vi "find_stage_goal_pose.vi"(6 "Pivot point (mm)":dbl[](array[numeric]), 7 "G^A: Goal (ASAP)":T1, 9 "L^A: Light pose (ASAP)":T1, 10 "E^B: current stage pose (base)":T1, 11 "O^A: base Orientation (ASAP)":T1) -> (1 "E'^B: goal pose (Base)":T1, 2 "t^O: translation ASAP -> base":T1, 3 "L^P: rotation of lights (Pivot)":T1)   [LabVIEW 2013]
uses:
  <vilib>/Analysis/Matrix/Datatypes/RealMatrix.ctl
  <vilib>/Analysis/baseanly.llb/Real A x B.vi
  <vilib>/Analysis/Matrix/Numeric/Conversions/Array To Matrix - RA.vi
  <vilib>/Analysis/NI_AALBase.lvlib
  <vilib>/Analysis/Matrix/NI_Matrix.lvlib
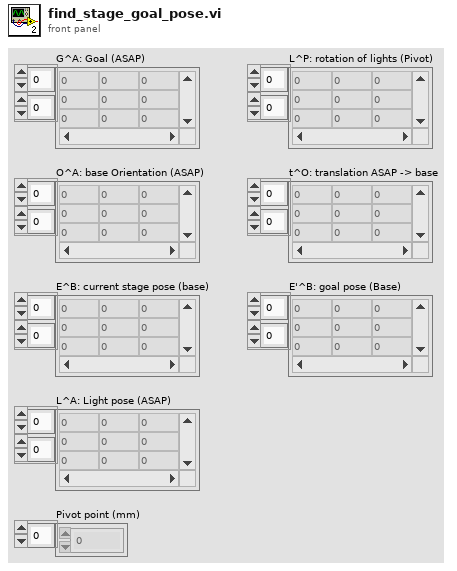
[diagram p1: front panel]
types:
  T1 = typedef "NI_Matrix.lvlib/RealMatrix.ctl" = dbl[][]
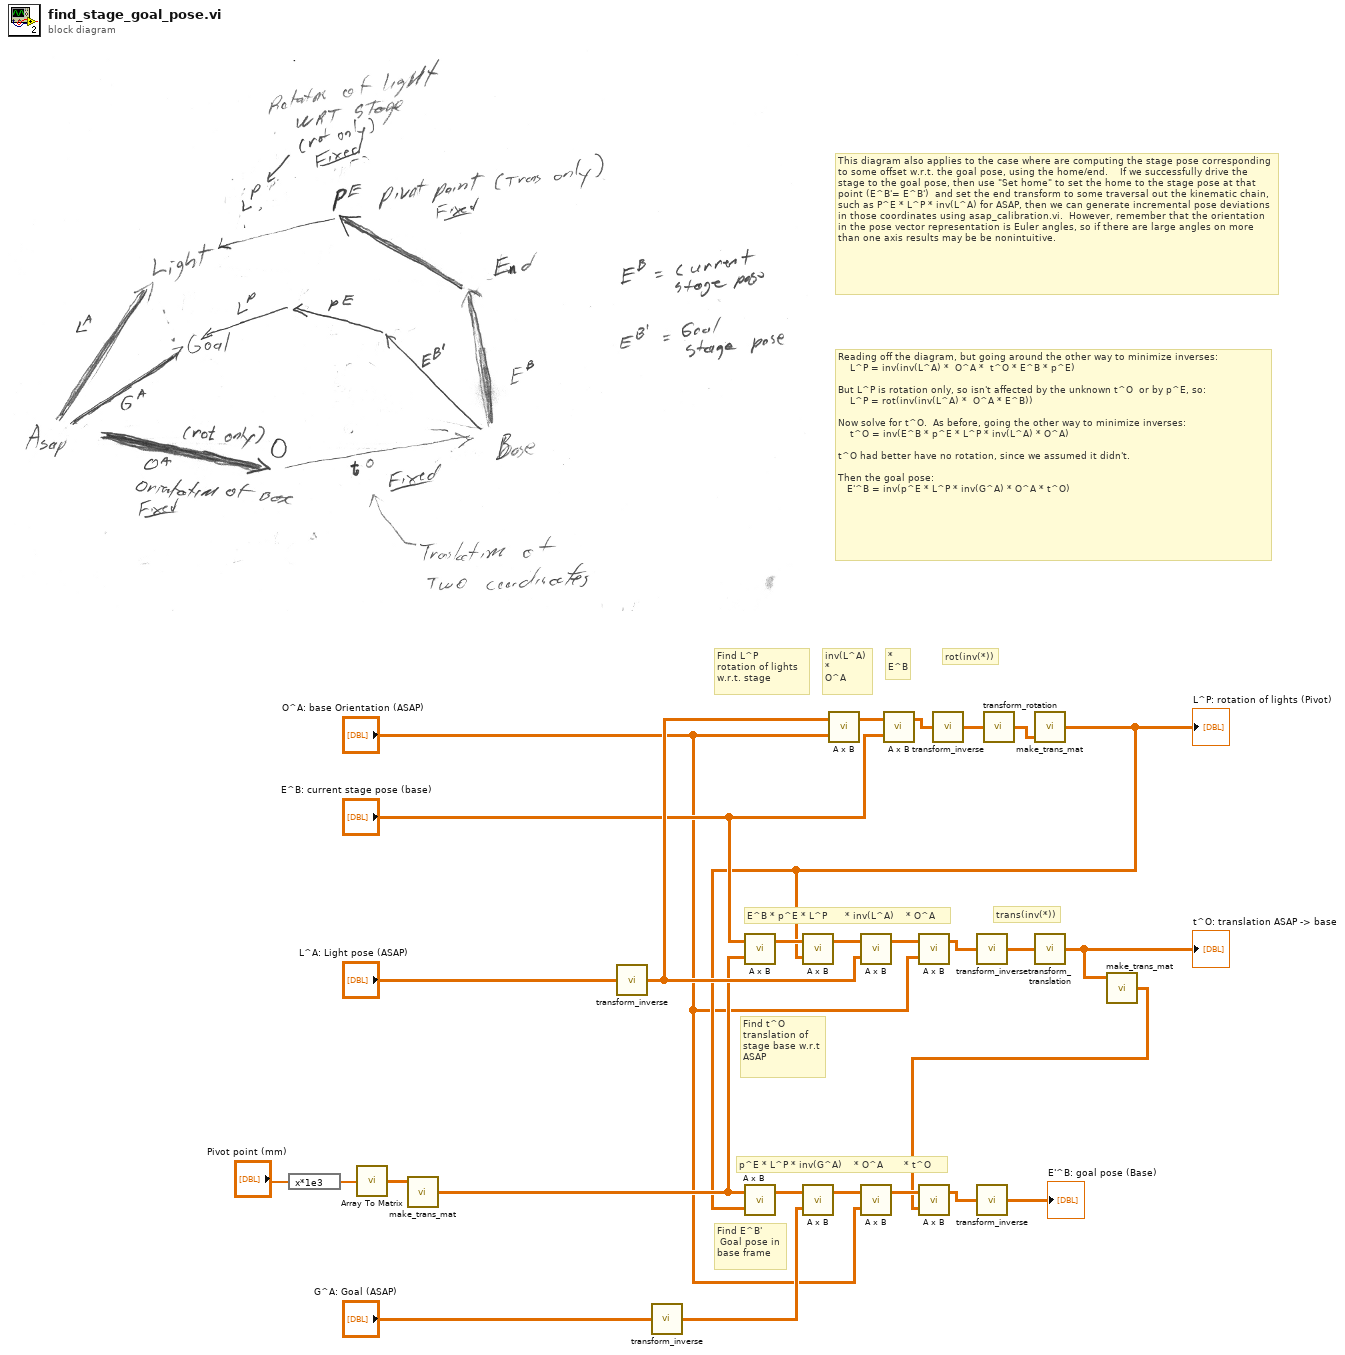
[diagram p0: block diagram]
diagram:
  # "This diagram also applies to the case where are computing the stage pose corresponding to some offset w.r.t. the goal pose, using the home/end.    If we successfully drive the stage to the goal pose, then use \"Set home\" to set the home to the stage pose at that point (E^B'= E^B')  and set the end transform to some traversal out the kinematic chain, such as P^E * L^P * inv(L^A) for ASAP, then we can generate incremental pose deviations in those coordinates using asap_calibration.vi.  However, remember that the orientation in the pose vector representation is Euler angles, so if there are large angles on more than one axis results may be be nonintuitive."
  # "Find t^O\ntranslation of\nstage base w.r.t\nASAP"
  # "p^E * L^P * inv(G^A)    * O^A       * t^O"
  # "trans(inv(*))"
  # "E^B * p^E * L^P      * inv(L^A)    * O^A"
  # "rot(inv(*))"
  # "Reading off the diagram, but going around the other way to minimize inverses:\n    L^P = inv(inv(L^A) *  O^A *  t^O * E^B * p^E)\n\nBut L^P is rotation only, so isn't affected by the unknown t^O  or by p^E, so:\n    L^P = rot(inv(inv(L^A) *  O^A * E^B))\n\nNow solve for t^O.  As before, going the other way to minimize inverses:\n    t^O = inv(E^B * p^E * L^P * inv(L^A) * O^A)\n\nt^O had better have no rotation, since we assumed it didn't.\n\nThen the goal pose:\n   E'^B = inv(p^E * L^P * inv(G^A) * O^A * t^O)"
  # "inv(L^A)\n*\nO^A"
  # "*\nE^B"
  # "Find E^B'\n Goal pose in\nbase frame"
  # "Find L^P\nrotation of lights \nw.r.t. stage"
  n1 = expression code="x*1e3"("Pivot point (mm)") -> (w23:dbl[])
  n2 = call-poly <vilib>:"Array To Matrix.vi"("Real 1D Array"=w23) -> ("Real Matrix (Column Vector)"=w24:T1)
  n3 = call "make_trans_mat.vi"("Translation"=w24) -> ("Transform"=w6:T1)  [unwired: 4 in]
  n4 = call "transform_inverse.vi"("Transform"="L^A: Light pose (ASAP)") -> ("Inverse transform"=w15:T1)
  n5 = call "transform_inverse.vi"("Transform"="G^A: Goal (ASAP)") -> ("Inverse transform"=w4:T1)
  n6 = call-poly <vilib>:"A x B.vi"("B"=w6, "A"="E^B: current stage pose (base)") -> ("A x B"=w12:T1)  [unwired: 1 out]
  n7 = call-poly <vilib>:"A x B.vi"("B"="O^A: base Orientation (ASAP)", "A"=w15) -> ("A x B"=w20:T1)  [unwired: 1 out]
  n8 = call-poly <vilib>:"A x B.vi"("B"="E^B: current stage pose (base)", "A"=w20) -> ("A x B"=w19:T1)  [unwired: 1 out]
  n9 = call "transform_inverse.vi"("Transform"=w19) -> ("Inverse transform"=w18:T1)
  n10 = call "transform_rotation.vi"("Transform"=w18) -> ("Rotation"=w25:T1)  [unwired: 4 in]
  n11 = call "make_trans_mat.vi"("Rotation"=w25) -> ("Transform"=w5:T1)  [unwired: 4 in]
  "L^P: rotation of lights (Pivot)" <- w5
  n12 = call-poly <vilib>:"A x B.vi"("B"=w5, "A"=w6) -> ("A x B"=w9:T1)  [unwired: 1 out]
  n13 = call-poly <vilib>:"A x B.vi"("B"=w5, "A"=w12) -> ("A x B"=w16:T1)  [unwired: 1 out]
  n14 = call-poly <vilib>:"A x B.vi"("B"=w4, "A"=w9) -> ("A x B"=w7:T1)  [unwired: 1 out]
  n15 = call-poly <vilib>:"A x B.vi"("B"=w15, "A"=w16) -> ("A x B"=w14:T1)  [unwired: 1 out]
  n16 = call-poly <vilib>:"A x B.vi"("B"="O^A: base Orientation (ASAP)", "A"=w7) -> ("A x B"=w8:T1)  [unwired: 1 out]
  n17 = call-poly <vilib>:"A x B.vi"("B"="O^A: base Orientation (ASAP)", "A"=w14) -> ("A x B"=w11:T1)  [unwired: 1 out]
  n18 = call "transform_inverse.vi"("Transform"=w11) -> ("Inverse transform"=w10:T1)
  n19 = call "transform_translation.vi"("Transform"=w10) -> ("Translation"=w26:T1)  [unwired: 4 in]
  "t^O: translation ASAP -> base" <- w26
  n20 = call "make_trans_mat.vi"("Translation"=w26) -> ("Transform"=w3:T1)  [unwired: 4 in]
  n21 = call-poly <vilib>:"A x B.vi"("B"=w3, "A"=w8) -> ("A x B"=w2:T1)  [unwired: 1 out]
  n22 = call "transform_inverse.vi"("Transform"=w2) -> ("Inverse transform"=→"E'^B: goal pose (Base)":T1)
